vi "InGaAs-GaAs QDSL-111221b- diff GIT - same T.vi"() -> ()   [LabVIEW 2011]
panel:
  out "step number  5":i32
  in  "Number of \nGrowth Steps 5":i32=10
  out "step number  4":i32
  in  "Number of \nGrowth Steps 4":i32=10
  out "step number  3":i32
  in  "Number of \nGrowth Steps 3":i32=10
  out "step number  2":i32
  in  "Number of \nGrowth Steps 2":i32=10
  in  "Indium Flow 2":dbl=55.0
  in  "Ga Flow 3":dbl=2.0
  in  "Ga Flow 2":dbl=2.41
  in  "Ga Flow 1":dbl=5.49
  in  "Indium Flow":dbl=44.0
  in  "Number of \nGrowth Steps":i32=10
  out "step number":i32
  in  "As_Gas Flow":dbl=3.4
  in  "Manifold H2 Flow":dbl=720.0
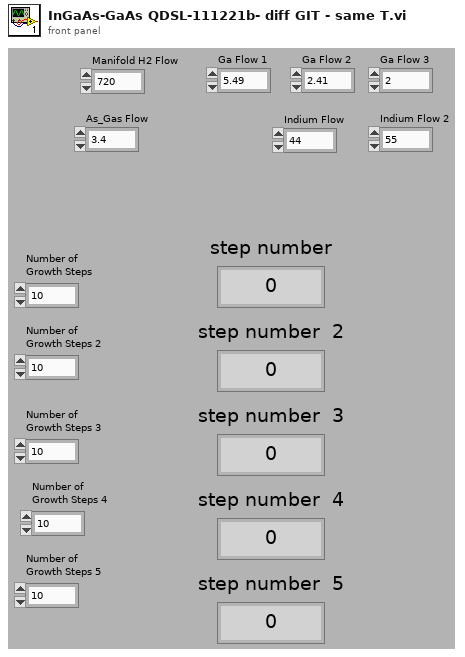
[diagram p1: front panel]
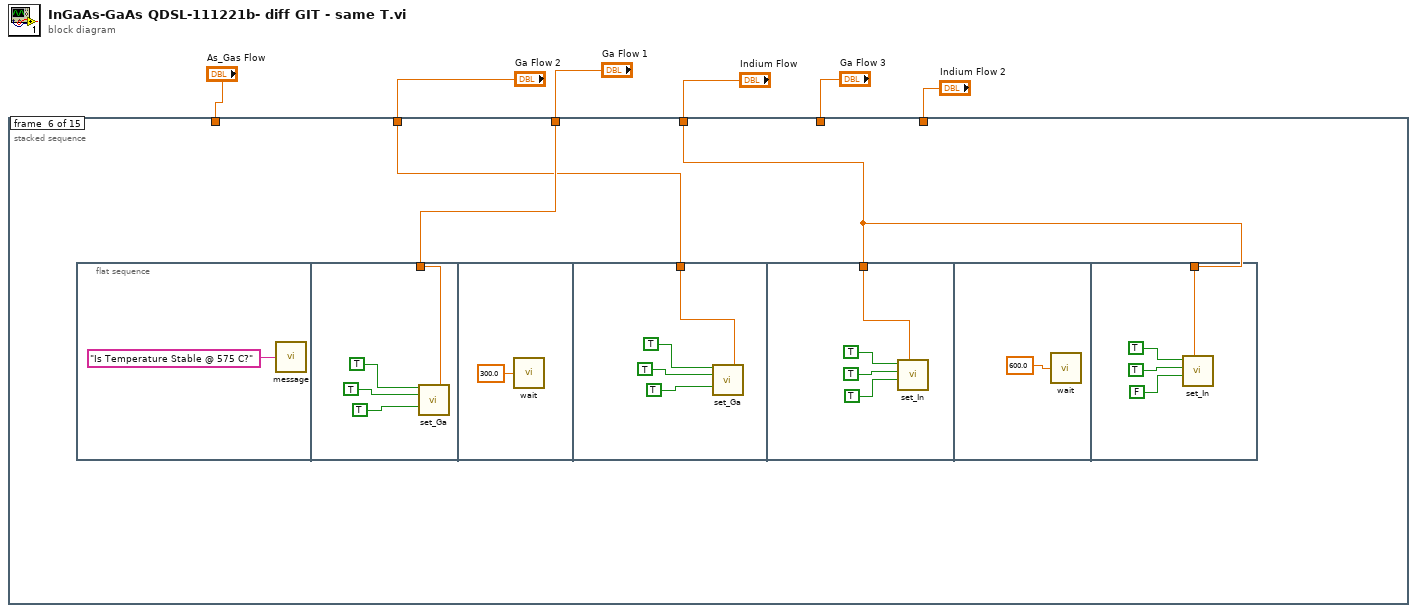
[diagram p0: block diagram]
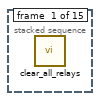
[diagram p2: hidden frame]
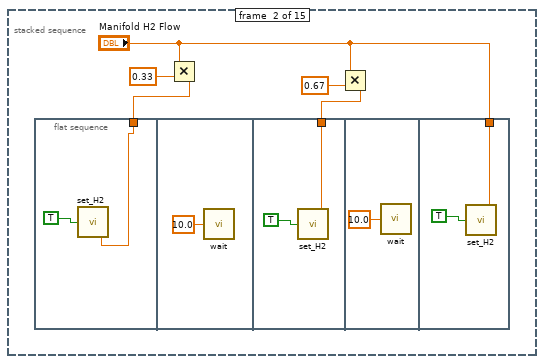
[diagram p3: hidden frame]
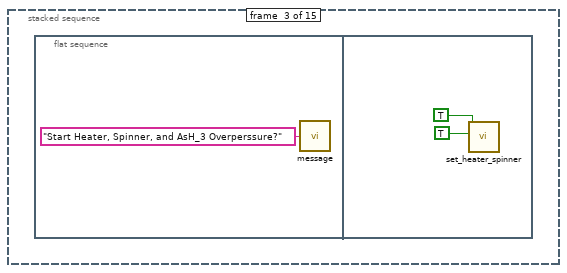
[diagram p4: hidden frame]
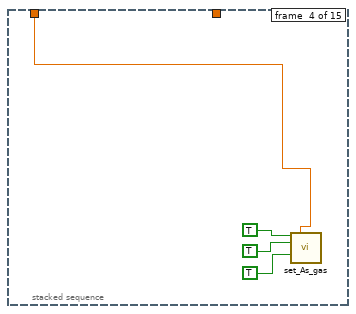
[diagram p5: hidden frame]
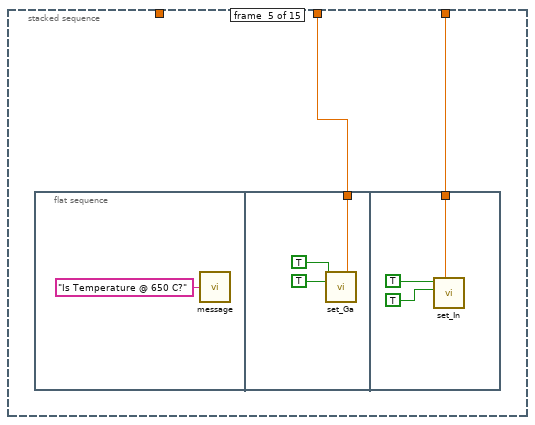
[diagram p6: hidden frame]
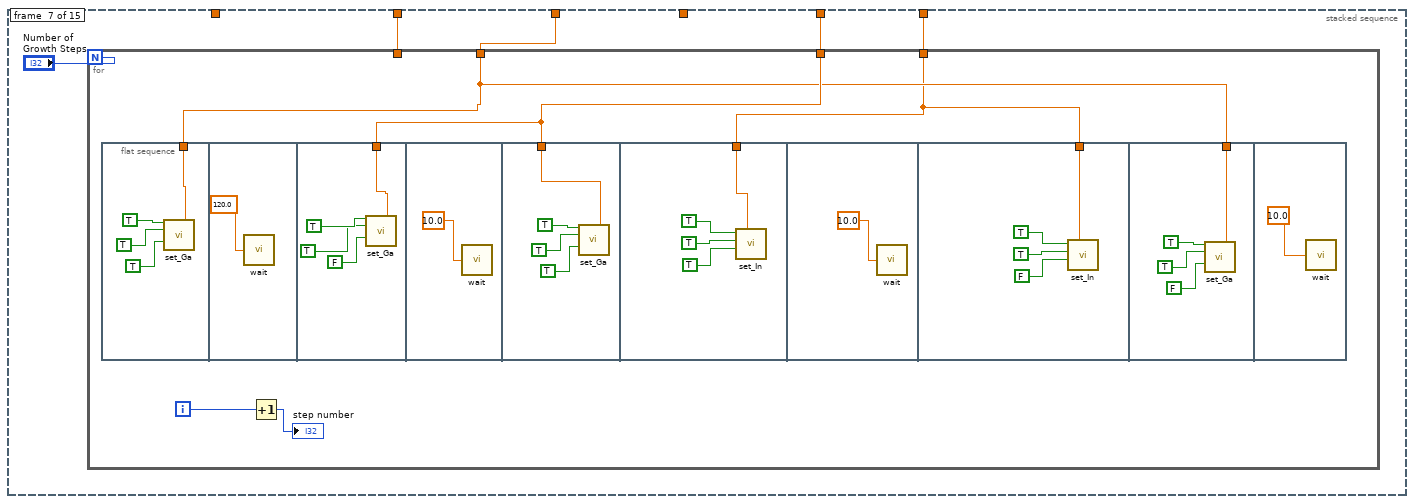
[diagram p7: hidden frame]
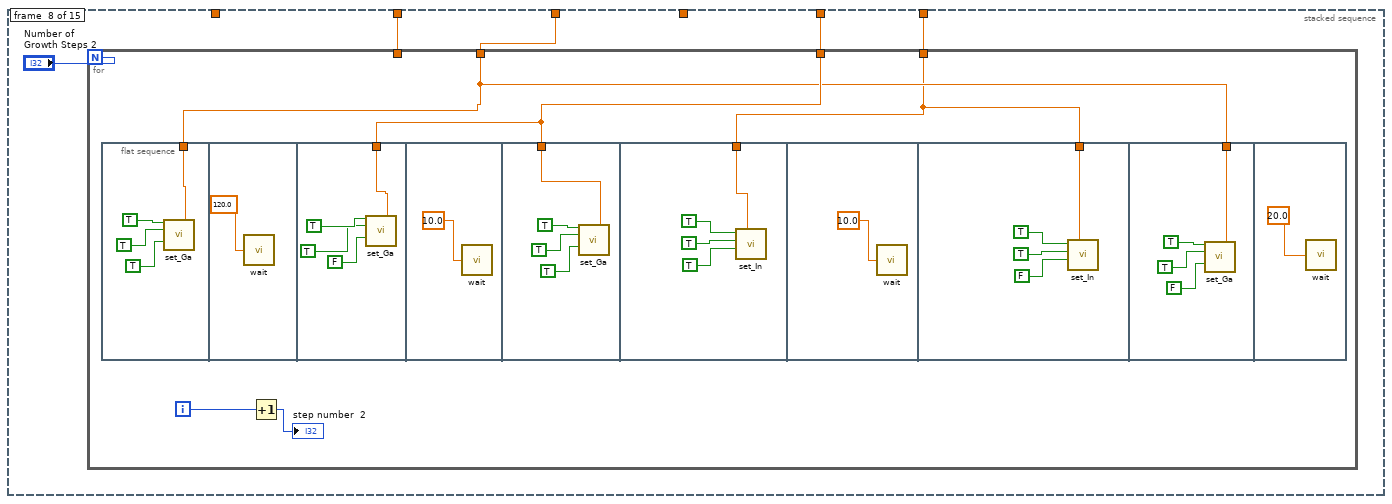
[diagram p8: hidden frame]
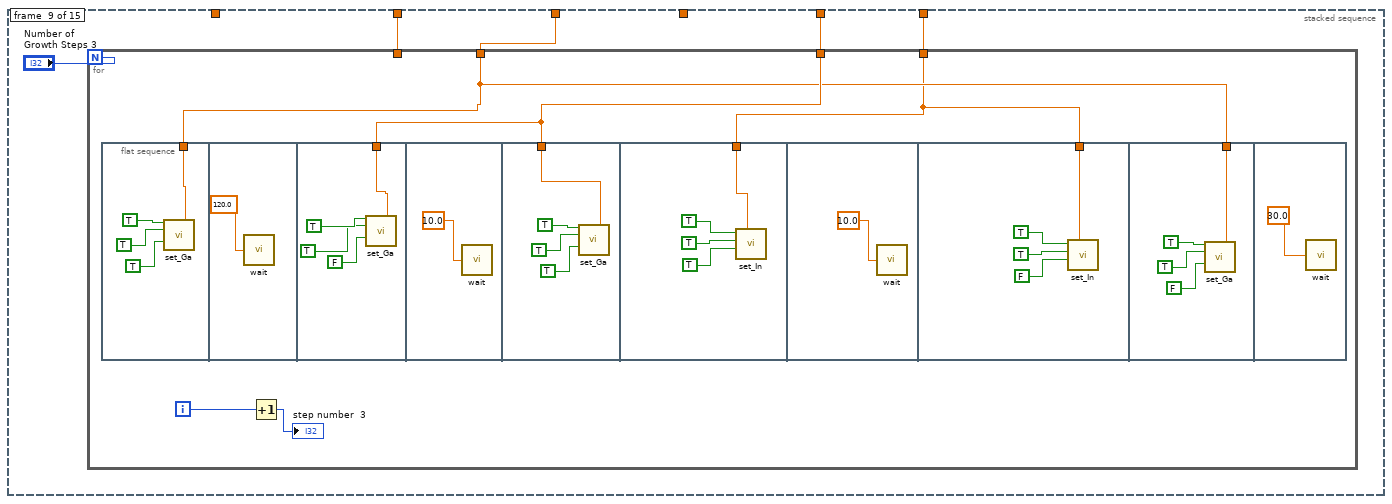
[diagram p9: hidden frame]
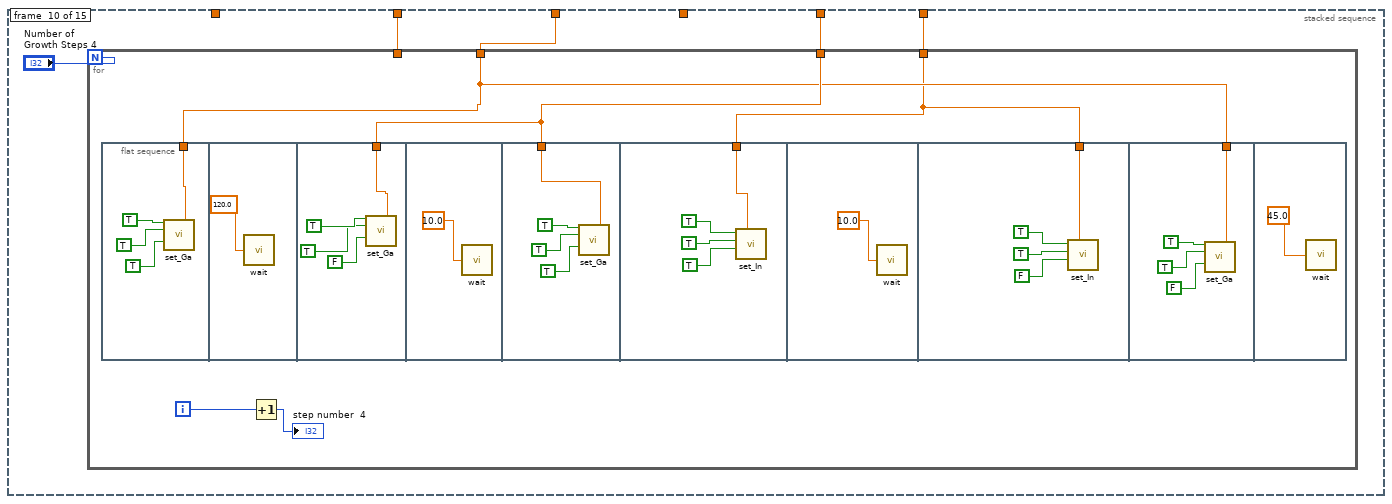
[diagram p10: hidden frame]
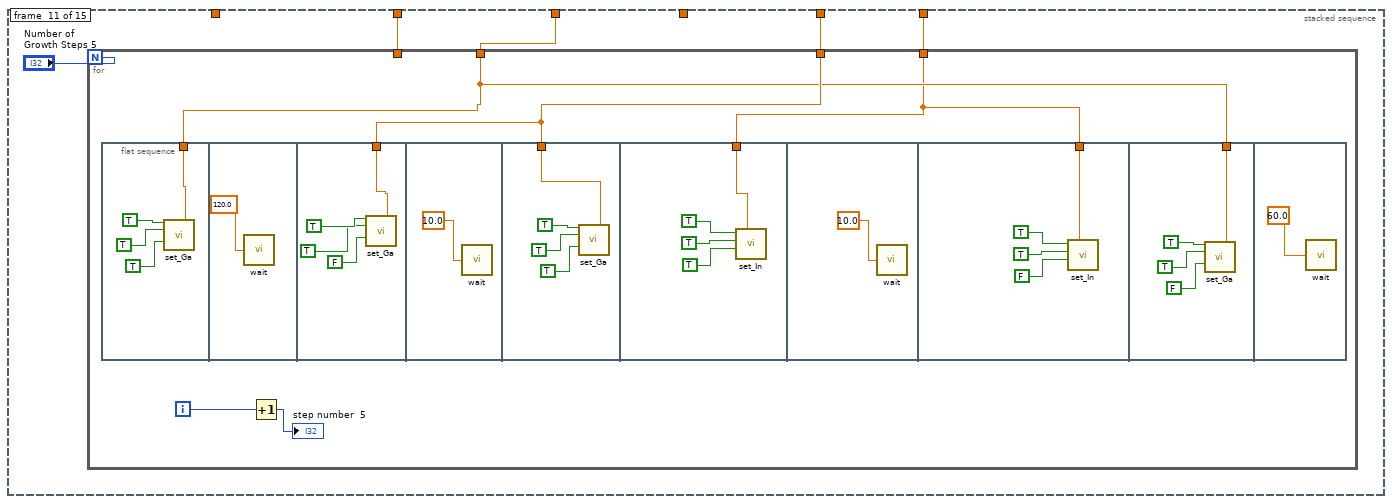
[diagram p11: hidden frame]
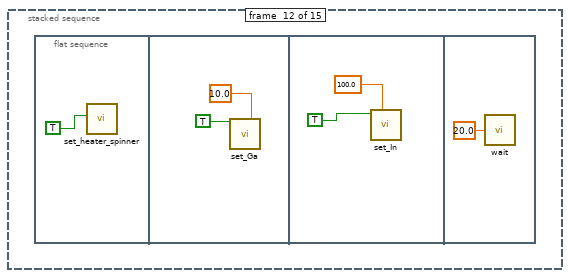
[diagram p12: hidden frame]
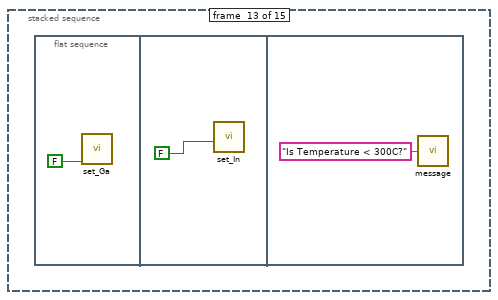
[diagram p13: hidden frame]
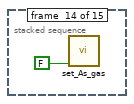
[diagram p14: hidden frame]
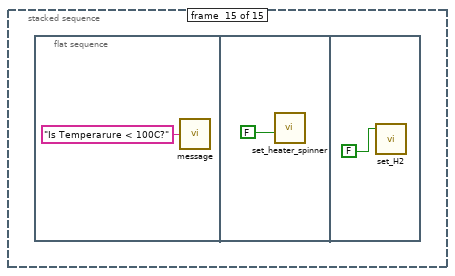
[diagram p15: hidden frame]
diagram:
  n1 = stacked-sequence {
    tunnel: "Ga Flow 1" -> [_ _ _ _ w28 w38 w61 w99 w137 w175 w213 _ _ _ _]
    tunnel: "As_Gas Flow" -> [_ _ _ w23 _ _ _ _ _ _ _ _ _ _ _]
    tunnel: "Indium Flow" -> [_ _ _ _ w27 w36 _ _ _ _ _ _ _ _ _]
    tunnel: "Ga Flow 2" -> [_ _ _ _ _ w37 w60 w98 w136 w174 w212 _ _ _ _]
    tunnel: "Ga Flow 3" -> [_ _ _ _ _ _ w59 w97 w135 w173 w211 _ _ _ _]
    tunnel: "Indium Flow 2" -> [_ _ _ _ _ _ w58 w96 w134 w172 w210 _ _ _ _]
    frame #0 {
      n2 = call "clear_all_relays.vi"() -> ()  [unwired: 2 out]
    }
    frame #1 {
      n3 = flat-sequence {
        tunnel: w11 -> [w12]
        tunnel: w9 -> [w15]
        tunnel: "Manifold H2 Flow" -> [w18]
        frame #0 {
          n4 = call "set_H2.vi"("Manifold H2 Flow"=w12, "H2 Active"=TRUE) -> ()  [unwired: 2 in, 2 out]
        }
        frame #1 {
          n5 = call "wait.vi"("Wait (s)"=10.0) -> ()
        }
        frame #2 {
          n6 = call "set_H2.vi"("Manifold H2 Flow"=w15, "H2 Active"=TRUE) -> ()  [unwired: 2 in, 2 out]
        }
        frame #3 {
          n7 = call "wait.vi"("Wait (s)"=10.0) -> ()
        }
        frame #4 {
          n8 = call "set_H2.vi"("Manifold H2 Flow"=w18, "H2 Active"=TRUE) -> ()  [unwired: 2 in, 2 out]
        }
      }
      n9 = Multiply(x="Manifold H2 Flow", y=0.33) -> (x*y=w11:dbl)
      n10 = Multiply(x="Manifold H2 Flow", y=0.67) -> (x*y=w9:dbl)
    }
    frame #2 {
      n11 = flat-sequence {
        frame #0 {
          n12 = call "message.vi"("message"="Start Heater, Spinner, and AsH_3 Overperssure?") -> ()
        }
        frame #1 {
          n13 = call "set_heater_spinner.vi"("Spinner"=TRUE, "Heater"=TRUE) -> ()  [unwired: 1 in, 7 out]
        }
      }
    }
    frame #3 {
      n14 = call "set_As_gas.vi"("As_Gas Active"=TRUE, "As_Gas Flow"=w23, "As_Gas In"=TRUE, "As_Gas Run"=TRUE) -> ()  [unwired: 2 in, 10 out]
    }
    frame #4 {
      n15 = flat-sequence {
        tunnel: w28 -> [w30]
        tunnel: w27 -> [w33]
        frame #0 {
          n16 = call "message.vi"("message"="Is Temperature @ 650 C?") -> ()
        }
        frame #1 {
          n17 = call "set_Ga.vi"("Ga Active"=TRUE, "Ga Flow 1"=w30, "Ga Bubbler"=TRUE) -> ()  [unwired: 5 in, 8 out]
        }
        frame #2 {
          n18 = call "set_In.vi"("Indium Flow"=w33, "In Bubbler"=TRUE ("Ga Bubbler"), "In Active"=TRUE ("Ga Active")) -> ()  [unwired: 2 in, 5 out]
        }
      }
    }
    frame #5 {
      n19 = flat-sequence {
        tunnel: w38 -> [w40]
        tunnel: w37 -> [w45]
        tunnel: w36 -> [w49]
        tunnel: w36 -> [w54]
        frame #0 {
          n20 = call "message.vi"("message"="Is Temperature Stable @ 575 C?") -> ()
        }
        frame #1 {
          n21 = call "set_Ga.vi"("Ga Active"=TRUE ("P_Gas Active"), "Ga Flow 1"=w40, "Ga Bubbler"=TRUE ("P_Gas In"), "Ga Run"=TRUE ("P_Gas Run")) -> ()  [unwired: 4 in, 8 out]
        }
        frame #2 {
          n22 = call "wait.vi"("Wait (s)"=300.0) -> ()
        }
        frame #3 {
          n23 = call "set_Ga.vi"("Ga Active"=TRUE ("P_Gas Active"), "Ga Flow 1"=w45, "Ga Bubbler"=TRUE ("P_Gas In"), "Ga Run"=TRUE ("P_Gas Run")) -> ()  [unwired: 4 in, 8 out]
        }
        frame #4 {
          n24 = call "set_In.vi"("Indium Flow"=w49, "In Run"=TRUE ("P_Gas Run"), "In Bubbler"=TRUE ("P_Gas In"), "In Active"=TRUE ("P_Gas Active")) -> ()  [unwired: 1 in, 5 out]
        }
        frame #5 {
          n25 = call "wait.vi"("Wait (s)"=600.0) -> ()
        }
        frame #6 {
          n26 = call "set_In.vi"("Indium Flow"=w54, "In Run"=FALSE ("P_Gas Run"), "In Bubbler"=TRUE ("P_Gas In"), "In Active"=TRUE ("P_Gas Active")) -> ()  [unwired: 1 in, 5 out]
        }
      }
    }
    frame #6 {
      n27 = for {
        N: "Number of \nGrowth Steps" -> [_]
        tunnel: w61 -> [w64]
        tunnel: w60 -> [_]
        tunnel: w59 -> [w65]
        tunnel: w58 -> [w63]
        i -> [w66]
        n28 = flat-sequence {
          tunnel: w64 -> [w68]
          tunnel: w65 -> [w73]
          tunnel: w65 -> [w78]
          tunnel: w63 -> [w82]
          tunnel: w63 -> [w87]
          tunnel: w64 -> [w91]
          frame #0 {
            n29 = call "set_Ga.vi"("Ga Active"=TRUE ("P_Gas Active"), "Ga Flow 1"=w68, "Ga Bubbler"=TRUE ("P_Gas In"), "Ga Run"=TRUE ("P_Gas Run")) -> ()  [unwired: 4 in, 8 out]
          }
          frame #1 {
            n30 = call "wait.vi"("Wait (s)"=120.0) -> ()
          }
          frame #2 {
            n31 = call "set_Ga.vi"("Ga Active"=TRUE ("P_Gas Active"), "Ga Flow 1"=w73, "Ga Bubbler"=TRUE ("P_Gas In"), "Ga Run"=FALSE ("P_Gas Run")) -> ()  [unwired: 4 in, 8 out]
          }
          frame #3 {
            n32 = call "wait.vi"("Wait (s)"=10.0) -> ()
          }
          frame #4 {
            n33 = call "set_Ga.vi"("Ga Active"=TRUE ("P_Gas Active"), "Ga Flow 1"=w78, "Ga Bubbler"=TRUE ("P_Gas In"), "Ga Run"=TRUE ("P_Gas Run")) -> ()  [unwired: 4 in, 8 out]
          }
          frame #5 {
            n34 = call "set_In.vi"("Indium Flow"=w82, "In Run"=TRUE ("P_Gas Run"), "In Bubbler"=TRUE ("P_Gas In"), "In Active"=TRUE ("P_Gas Active")) -> ()  [unwired: 1 in, 5 out]
          }
          frame #6 {
            n35 = call "wait.vi"("Wait (s)"=10.0) -> ()
          }
          frame #7 {
            n36 = call "set_In.vi"("Indium Flow"=w87, "In Run"=FALSE ("P_Gas Run"), "In Bubbler"=TRUE ("P_Gas In"), "In Active"=TRUE ("P_Gas Active")) -> ()  [unwired: 1 in, 5 out]
          }
          frame #8 {
            n37 = call "set_Ga.vi"("Ga Active"=TRUE ("P_Gas Active"), "Ga Flow 1"=w91, "Ga Bubbler"=TRUE ("P_Gas In"), "Ga Run"=FALSE ("P_Gas Run")) -> ()  [unwired: 4 in, 8 out]
          }
          frame #9 {
            n38 = call "wait.vi"("Wait (s)"=10.0) -> ()
          }
        }
        n39 = Increment(x=w66) -> (x+1=→"step number":i32)
      }
    }
    frame #7 {
      n40 = for {
        N: "Number of \nGrowth Steps 2" -> [_]
        tunnel: w99 -> [w102]
        tunnel: w98 -> [_]
        tunnel: w97 -> [w103]
        tunnel: w96 -> [w101]
        i -> [w104]
        n41 = flat-sequence {
          tunnel: w102 -> [w106]
          tunnel: w103 -> [w111]
          tunnel: w103 -> [w116]
          tunnel: w101 -> [w120]
          tunnel: w101 -> [w125]
          tunnel: w102 -> [w129]
          frame #0 {
            n42 = call "set_Ga.vi"("Ga Active"=TRUE ("P_Gas Active"), "Ga Flow 1"=w106, "Ga Bubbler"=TRUE ("P_Gas In"), "Ga Run"=TRUE ("P_Gas Run")) -> ()  [unwired: 4 in, 8 out]
          }
          frame #1 {
            n43 = call "wait.vi"("Wait (s)"=120.0) -> ()
          }
          frame #2 {
            n44 = call "set_Ga.vi"("Ga Active"=TRUE ("P_Gas Active"), "Ga Flow 1"=w111, "Ga Bubbler"=TRUE ("P_Gas In"), "Ga Run"=FALSE ("P_Gas Run")) -> ()  [unwired: 4 in, 8 out]
          }
          frame #3 {
            n45 = call "wait.vi"("Wait (s)"=10.0) -> ()
          }
          frame #4 {
            n46 = call "set_Ga.vi"("Ga Active"=TRUE ("P_Gas Active"), "Ga Flow 1"=w116, "Ga Bubbler"=TRUE ("P_Gas In"), "Ga Run"=TRUE ("P_Gas Run")) -> ()  [unwired: 4 in, 8 out]
          }
          frame #5 {
            n47 = call "set_In.vi"("Indium Flow"=w120, "In Run"=TRUE ("P_Gas Run"), "In Bubbler"=TRUE ("P_Gas In"), "In Active"=TRUE ("P_Gas Active")) -> ()  [unwired: 1 in, 5 out]
          }
          frame #6 {
            n48 = call "wait.vi"("Wait (s)"=10.0) -> ()
          }
          frame #7 {
            n49 = call "set_In.vi"("Indium Flow"=w125, "In Run"=FALSE ("P_Gas Run"), "In Bubbler"=TRUE ("P_Gas In"), "In Active"=TRUE ("P_Gas Active")) -> ()  [unwired: 1 in, 5 out]
          }
          frame #8 {
            n50 = call "set_Ga.vi"("Ga Active"=TRUE ("P_Gas Active"), "Ga Flow 1"=w129, "Ga Bubbler"=TRUE ("P_Gas In"), "Ga Run"=FALSE ("P_Gas Run")) -> ()  [unwired: 4 in, 8 out]
          }
          frame #9 {
            n51 = call "wait.vi"("Wait (s)"=20.0) -> ()
          }
        }
        n52 = Increment(x=w104) -> (x+1=→"step number  2":i32)
      }
    }
    frame #8 {
      n53 = for {
        N: "Number of \nGrowth Steps 3" -> [_]
        tunnel: w137 -> [w140]
        tunnel: w136 -> [_]
        tunnel: w135 -> [w141]
        tunnel: w134 -> [w139]
        i -> [w142]
        n54 = flat-sequence {
          tunnel: w140 -> [w144]
          tunnel: w141 -> [w149]
          tunnel: w141 -> [w154]
          tunnel: w139 -> [w158]
          tunnel: w139 -> [w163]
          tunnel: w140 -> [w167]
          frame #0 {
            n55 = call "set_Ga.vi"("Ga Active"=TRUE ("P_Gas Active"), "Ga Flow 1"=w144, "Ga Bubbler"=TRUE ("P_Gas In"), "Ga Run"=TRUE ("P_Gas Run")) -> ()  [unwired: 4 in, 8 out]
          }
          frame #1 {
            n56 = call "wait.vi"("Wait (s)"=120.0) -> ()
          }
          frame #2 {
            n57 = call "set_Ga.vi"("Ga Active"=TRUE ("P_Gas Active"), "Ga Flow 1"=w149, "Ga Bubbler"=TRUE ("P_Gas In"), "Ga Run"=FALSE ("P_Gas Run")) -> ()  [unwired: 4 in, 8 out]
          }
          frame #3 {
            n58 = call "wait.vi"("Wait (s)"=10.0) -> ()
          }
          frame #4 {
            n59 = call "set_Ga.vi"("Ga Active"=TRUE ("P_Gas Active"), "Ga Flow 1"=w154, "Ga Bubbler"=TRUE ("P_Gas In"), "Ga Run"=TRUE ("P_Gas Run")) -> ()  [unwired: 4 in, 8 out]
          }
          frame #5 {
            n60 = call "set_In.vi"("Indium Flow"=w158, "In Run"=TRUE ("P_Gas Run"), "In Bubbler"=TRUE ("P_Gas In"), "In Active"=TRUE ("P_Gas Active")) -> ()  [unwired: 1 in, 5 out]
          }
          frame #6 {
            n61 = call "wait.vi"("Wait (s)"=10.0) -> ()
          }
          frame #7 {
            n62 = call "set_In.vi"("Indium Flow"=w163, "In Run"=FALSE ("P_Gas Run"), "In Bubbler"=TRUE ("P_Gas In"), "In Active"=TRUE ("P_Gas Active")) -> ()  [unwired: 1 in, 5 out]
          }
          frame #8 {
            n63 = call "set_Ga.vi"("Ga Active"=TRUE ("P_Gas Active"), "Ga Flow 1"=w167, "Ga Bubbler"=TRUE ("P_Gas In"), "Ga Run"=FALSE ("P_Gas Run")) -> ()  [unwired: 4 in, 8 out]
          }
          frame #9 {
            n64 = call "wait.vi"("Wait (s)"=30.0) -> ()
          }
        }
        n65 = Increment(x=w142) -> (x+1=→"step number  3":i32)
      }
    }
    frame #9 {
      n66 = for {
        N: "Number of \nGrowth Steps 4" -> [_]
        tunnel: w175 -> [w178]
        tunnel: w174 -> [_]
        tunnel: w173 -> [w179]
        tunnel: w172 -> [w177]
        i -> [w180]
        n67 = flat-sequence {
          tunnel: w178 -> [w182]
          tunnel: w179 -> [w187]
          tunnel: w179 -> [w192]
          tunnel: w177 -> [w196]
          tunnel: w177 -> [w201]
          tunnel: w178 -> [w205]
          frame #0 {
            n68 = call "set_Ga.vi"("Ga Active"=TRUE ("P_Gas Active"), "Ga Flow 1"=w182, "Ga Bubbler"=TRUE ("P_Gas In"), "Ga Run"=TRUE ("P_Gas Run")) -> ()  [unwired: 4 in, 8 out]
          }
          frame #1 {
            n69 = call "wait.vi"("Wait (s)"=120.0) -> ()
          }
          frame #2 {
            n70 = call "set_Ga.vi"("Ga Active"=TRUE ("P_Gas Active"), "Ga Flow 1"=w187, "Ga Bubbler"=TRUE ("P_Gas In"), "Ga Run"=FALSE ("P_Gas Run")) -> ()  [unwired: 4 in, 8 out]
          }
          frame #3 {
            n71 = call "wait.vi"("Wait (s)"=10.0) -> ()
          }
          frame #4 {
            n72 = call "set_Ga.vi"("Ga Active"=TRUE ("P_Gas Active"), "Ga Flow 1"=w192, "Ga Bubbler"=TRUE ("P_Gas In"), "Ga Run"=TRUE ("P_Gas Run")) -> ()  [unwired: 4 in, 8 out]
          }
          frame #5 {
            n73 = call "set_In.vi"("Indium Flow"=w196, "In Run"=TRUE ("P_Gas Run"), "In Bubbler"=TRUE ("P_Gas In"), "In Active"=TRUE ("P_Gas Active")) -> ()  [unwired: 1 in, 5 out]
          }
          frame #6 {
            n74 = call "wait.vi"("Wait (s)"=10.0) -> ()
          }
          frame #7 {
            n75 = call "set_In.vi"("Indium Flow"=w201, "In Run"=FALSE ("P_Gas Run"), "In Bubbler"=TRUE ("P_Gas In"), "In Active"=TRUE ("P_Gas Active")) -> ()  [unwired: 1 in, 5 out]
          }
          frame #8 {
            n76 = call "set_Ga.vi"("Ga Active"=TRUE ("P_Gas Active"), "Ga Flow 1"=w205, "Ga Bubbler"=TRUE ("P_Gas In"), "Ga Run"=FALSE ("P_Gas Run")) -> ()  [unwired: 4 in, 8 out]
          }
          frame #9 {
            n77 = call "wait.vi"("Wait (s)"=45.0) -> ()
          }
        }
        n78 = Increment(x=w180) -> (x+1=→"step number  4":i32)
      }
    }
    frame #10 {
      n79 = for {
        N: "Number of \nGrowth Steps 5" -> [_]
        tunnel: w213 -> [w216]
        tunnel: w212 -> [_]
        tunnel: w211 -> [w217]
        tunnel: w210 -> [w215]
        i -> [w218]
        n80 = flat-sequence {
          tunnel: w216 -> [w220]
          tunnel: w217 -> [w225]
          tunnel: w217 -> [w230]
          tunnel: w215 -> [w234]
          tunnel: w215 -> [w239]
          tunnel: w216 -> [w243]
          frame #0 {
            n81 = call "set_Ga.vi"("Ga Active"=TRUE ("P_Gas Active"), "Ga Flow 1"=w220, "Ga Bubbler"=TRUE ("P_Gas In"), "Ga Run"=TRUE ("P_Gas Run")) -> ()  [unwired: 4 in, 8 out]
          }
          frame #1 {
            n82 = call "wait.vi"("Wait (s)"=120.0) -> ()
          }
          frame #2 {
            n83 = call "set_Ga.vi"("Ga Active"=TRUE ("P_Gas Active"), "Ga Flow 1"=w225, "Ga Bubbler"=TRUE ("P_Gas In"), "Ga Run"=FALSE ("P_Gas Run")) -> ()  [unwired: 4 in, 8 out]
          }
          frame #3 {
            n84 = call "wait.vi"("Wait (s)"=10.0) -> ()
          }
          frame #4 {
            n85 = call "set_Ga.vi"("Ga Active"=TRUE ("P_Gas Active"), "Ga Flow 1"=w230, "Ga Bubbler"=TRUE ("P_Gas In"), "Ga Run"=TRUE ("P_Gas Run")) -> ()  [unwired: 4 in, 8 out]
          }
          frame #5 {
            n86 = call "set_In.vi"("Indium Flow"=w234, "In Run"=TRUE ("P_Gas Run"), "In Bubbler"=TRUE ("P_Gas In"), "In Active"=TRUE ("P_Gas Active")) -> ()  [unwired: 1 in, 5 out]
          }
          frame #6 {
            n87 = call "wait.vi"("Wait (s)"=10.0) -> ()
          }
          frame #7 {
            n88 = call "set_In.vi"("Indium Flow"=w239, "In Run"=FALSE ("P_Gas Run"), "In Bubbler"=TRUE ("P_Gas In"), "In Active"=TRUE ("P_Gas Active")) -> ()  [unwired: 1 in, 5 out]
          }
          frame #8 {
            n89 = call "set_Ga.vi"("Ga Active"=TRUE ("P_Gas Active"), "Ga Flow 1"=w243, "Ga Bubbler"=TRUE ("P_Gas In"), "Ga Run"=FALSE ("P_Gas Run")) -> ()  [unwired: 4 in, 8 out]
          }
          frame #9 {
            n90 = call "wait.vi"("Wait (s)"=60.0) -> ()
          }
        }
        n91 = Increment(x=w218) -> (x+1=→"step number  5":i32)
      }
    }
    frame #11 {
      n92 = flat-sequence {
        frame #0 {
          n93 = call "set_heater_spinner.vi"("Spinner"=TRUE ("Ga Active")) -> ()  [unwired: 2 in, 7 out]
        }
        frame #1 {
          n94 = call "set_Ga.vi"("Ga Active"=TRUE, "Ga Flow 1"=10.0) -> ()  [unwired: 6 in, 8 out]
        }
        frame #2 {
          n95 = call "set_In.vi"("Indium Flow"=100.0 ("Aluminum Flow"), "In Active"=TRUE ("Ga Active")) -> ()  [unwired: 3 in, 5 out]
        }
        frame #3 {
          n96 = call "wait.vi"("Wait (s)"=20.0) -> ()
        }
      }
    }
    frame #12 {
      n97 = flat-sequence {
        frame #0 {
          n98 = call "set_Ga.vi"("Ga Remote"=FALSE) -> ()  [unwired: 7 in, 8 out]
        }
        frame #1 {
          n99 = call "set_In.vi"("In Run"=FALSE ("Ga Remote")) -> ()  [unwired: 4 in, 5 out]
        }
        frame #2 {
          n100 = call "message.vi"("message"="Is Temperature < 300C?") -> ()
        }
      }
    }
    frame #13 {
      n101 = call "set_As_gas.vi"("As_Gas Remote"=FALSE) -> ()  [unwired: 5 in, 10 out]
    }
    frame #14 {
      n102 = flat-sequence {
        frame #0 {
          n103 = call "message.vi"("message"="Is Temperarure < 100C?") -> ()
        }
        frame #1 {
          n104 = call "set_heater_spinner.vi"("Heater/Spinner Remote"=FALSE) -> ()  [unwired: 2 in, 7 out]
        }
        frame #2 {
          n105 = call "set_H2.vi"("H2N2 Remote"=FALSE) -> ()  [unwired: 3 in, 2 out]
        }
      }
    }
  }
